vi "Generate Measurement Server Internal.vi"() -> ()   [LabVIEW 2020]
uses:
  Generator/_Editor/MeasurementService Editor.lvlib
panel:
  in  "Debug - Leave Project Open? (F)":bool
  out "error out":errorcluster
  in  "error in (no error)":errorcluster
  # "Currently this VI assumes many things... Should consider implementing improvements to reduce assumptions\n\nAssumptions:\n1. The pre-existing virtual folder has been removed from the .lvproject\n-- could do this programmatically\n2. The pre-existing directory has been removed from disk\n-- could do this programmatically\n5. The project is not open when running the generator\n-- Could do this programmatically"
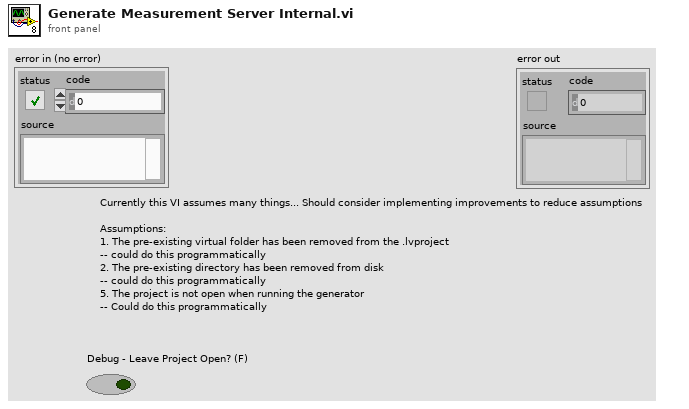
[diagram p1: front panel]
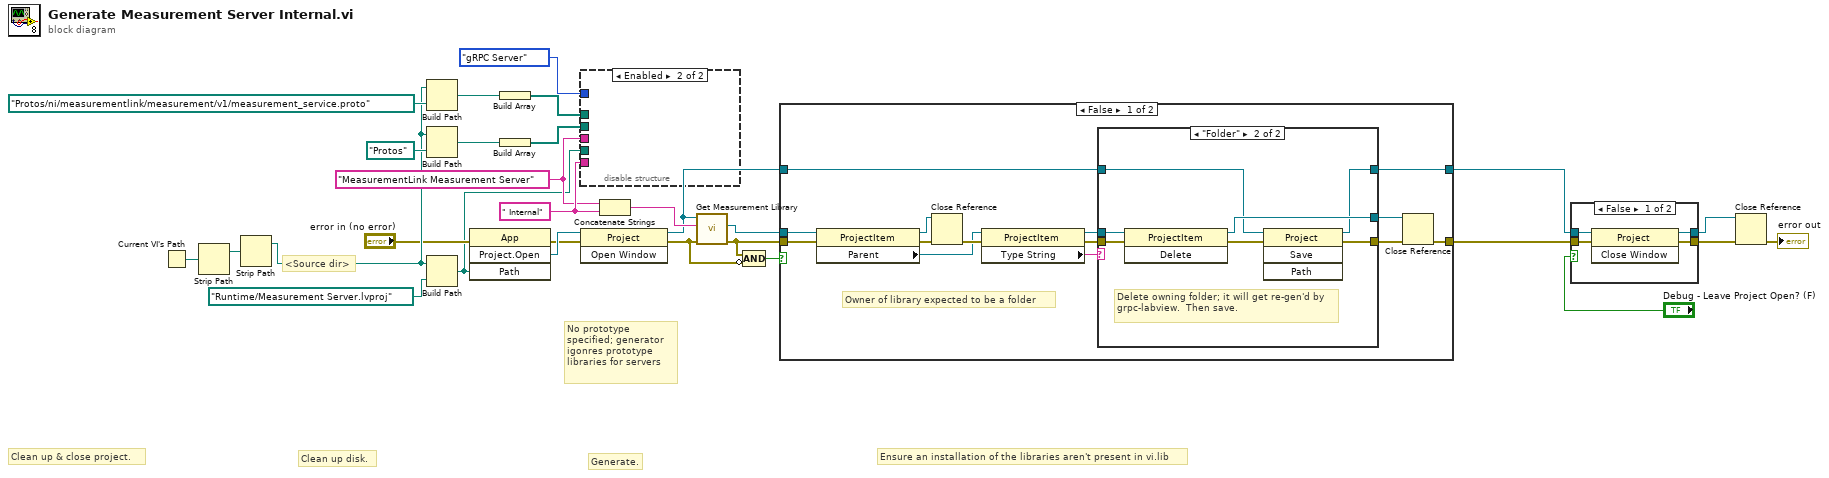
[diagram p0: block diagram]
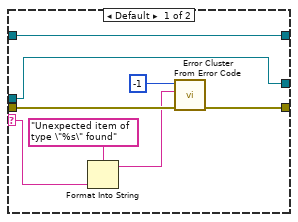
[diagram p2: hidden frame]
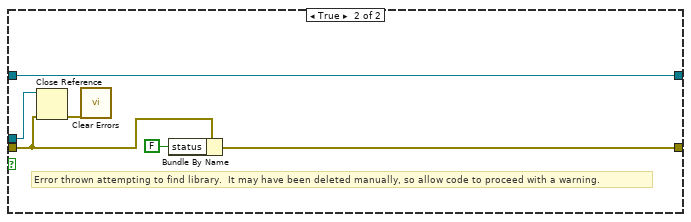
[diagram p3: hidden frame]
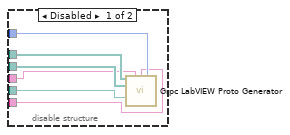
[diagram p5: hidden frame]
diagram:
  w19 = " Internal" ("Library Suffix")
  w18 = "MeasurementLink Measurement Server" ("Generated Library Name")
  # "Ensure an installation of the libraries aren't present in vi.lib"
  # "Generate."
  # "Clean up disk."
  # "Clean up & close project."
  # "No prototype specified; generator igonres prototype libraries for servers"
  # "<Source dir>"
  n1 = Current VI's Path() -> (path=w16:path)
  n2 = Strip Path(path=w16) -> (stripped path=w15:path)  [unwired: 1 out]
  n3 = Strip Path(path=w15) -> (stripped path=w22:path)  [unwired: 1 out]
  n4 = Build Path(base path=w22, name or relative path=path "Protos/ni/measurementlink/measurement/v1/measurement_service.proto" ("Proto File Path")) -> (appended path=w27:path)
  n5 = Build Path(base path=w22, name or relative path=path "Protos" ("Proto File Path")) -> (appended path=w24:path)
  n6 = Build Path(base path=w22, name or relative path=path "Runtime/Measurement Server.lvproj" ("Target Project")) -> (appended path=w12:path)
  n7 = invoke class="App" method="Project.Open"(error in="error in (no error)", "Path"=w12) -> (error out=w13:errorcluster, "Project:Open"=w14:refnum<vi>)  [unwired: 2 in, 2 out]
  n8 = Build Array(w27) -> (w26:path[])
  n9 = Build Array(w24) -> (w23:path[])
  n10 = disable-structure shown="Enabled" {
    disable-tunnel: enum16{"gRPC Server", "gRPC Client", "Both"}."gRPC Server" ("Generate") -> [w35 _]
    disable-tunnel: w12 -> [w34 _]
    disable-tunnel: w26 -> [w33 _]
    disable-tunnel: w23 -> [w32 _]
    disable-tunnel: w19 -> [w31 _]
    disable-tunnel: w18 -> [w30 _]
    frame Disabled {
      n11 = call "Grpc LabVIEW Proto Generator.vi"("Proto File Path"=w33, "Generated Library Name"=w30, "Library Suffix"=w31, "Generate"=w35, "Import Paths"=w32, "Target Project"=w34) -> ()  [unwired: 9 in, 1 out]
    }
    frame Enabled {
    }
  }
  n12 = invoke class="Project" method="Open Window"(reference=w14, error in=w13) -> (reference out=w1:refnum<vi>, error out=w5:errorcluster)  [unwired: 1 in, 1 out]
  n13 = Concatenate Strings(w18, w19) -> (w2:string)
  n14 = call "Get Measurement Library.vi"("error in (no error)"=w5, "Measurement Service Name"=w2, "Project in"=w1) -> ("error out"=w4:errorcluster, "Measurement Library Item"=w3:refnum<vi>)  [unwired: 7 in]
  n15 = Compound Arithmetic op=AND(w4, invert w5) -> (w6:bool)
  n16 = case shown="False" w6 {
    tunnel: w3 -> [w48 w67]
    tunnel: w1 -> [w41 w68]
    tunnel: [w38 w68] -> w11
    tunnel: [w37 w70] -> w10
    tunnel: w4 -> [w36 w66]
    frame False {
      # "Owner of library expected to be a folder"
      n17 = property class="ProjectItem"(reference=w48, error in=w36) -> (reference out=w47:refnum<vi>, error out=w49:errorcluster, "Parent"=w45:refnum<vi>)
      n18 = Close Reference(reference=w47, error in (no error)=w49) -> (error out=w46:errorcluster)
      n19 = property class="ProjectItem"(reference=w45, error in=w46) -> (reference out=w42:refnum<vi>, error out=w43:errorcluster, "Type String"=w44:string)
      n20 = case shown="\"Folder\"" w44 {
        selector: w44 -> [w54 _]
        tunnel: w43 -> [w57 w64]
        tunnel: w42 -> [w51 w63]
        tunnel: [w56 w60] -> w40
        tunnel: w41 -> [w50 w59]
        tunnel: [w50 w58] -> w38
        tunnel: [w51 w62] -> w39
        frame Default {
          n21 = Format Into String(format string="Unexpected item of type \"%s\" found", w54) -> (resulting string=w53:string)  [unwired: 2 in, 1 out]
          n22 = call <vilib>:"Error Cluster From Error Code.vi"("error in (no error)"=w57, "error message (\"\")"=w53, "error code (0)"=-1) -> ("error out"=w56:errorcluster)  [unwired: 6 in]
        }
        frame "Folder" {
          # "Delete owning folder; it will get re-gen'd by grpc-labview.  Then save."
          n23 = invoke class="ProjectItem" method="Delete"(reference=w63, error in=w64) -> (reference out=w62:refnum<vi>, error out=w61:errorcluster)  [unwired: 1 in, 1 out]
          n24 = invoke class="Project" method="Save"(reference=w59, error in=w61) -> (reference out=w58:refnum<vi>, error out=w60:errorcluster)  [unwired: 2 in, 2 out]
        }
      }
      n25 = Close Reference(reference=w39, error in (no error)=w40) -> (error out=w37:errorcluster)
    }
    frame True {
      # "Error thrown attempting to find library.  It may have been deleted manually, so allow code to proceed with a warning."
      n26 = Close Reference(reference=w67, error in (no error)=w66) -> (error out=w65:errorcluster)
      n27 = call <vilib>:"Clear Errors.vi"("error in (no error)"=w65) -> ()  [unwired: 5 in, 2 out]
      n28 = Bundle By Name(cluster=w66, "status"=FALSE) -> (w70:errorcluster)
    }
  }
  n29 = case shown="False" "Debug - Leave Project Open? (F)" {
    tunnel: w11 -> [w74 w75]
    tunnel: w10 -> [w73 w76]
    tunnel: [w72 w76] -> w9
    tunnel: [w71 w75] -> w8
    frame False {
      n30 = invoke class="Project" method="Close Window"(reference=w74, error in=w73) -> (reference out=w71:refnum<vi>, error out=w72:errorcluster)  [unwired: 1 in, 1 out]
    }
    frame True {
    }
  }
  n31 = Close Reference(reference=w8, error in (no error)=w9) -> (error out=→"error out":errorcluster)
